vi "DAQ.Calibrate.vi"(8 "error in (no error)":errorcluster, 11 "Lockin.DAQ in":refnum<class "Instrument.DAQ.lvclass">) -> (0 "error out":errorcluster, 3 "Lockin.DAQ out":refnum<class "Instrument.DAQ.lvclass">)   [LabVIEW 2019, in "Instrument.Lockin.lvlib" / "Instrument.DAQ.lvclass"]
uses:
  Instrument.DAQ.lvclass
  DAQmx/typedefs/DAQmx.Commands--enum.ctl
  Instrument.DAQ.lvclass/Instrument.DAQ.ctl
  DAQmx/DAQmx.lvclass
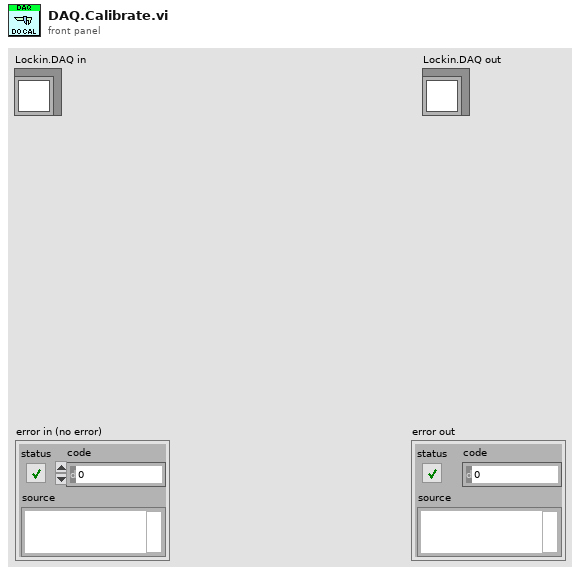
[diagram p1: front panel]
types:
  T1 = typedef "DAQmx.lvclass/DAQmx.Commands--enum.ctl" = enum16{"idle", "start", "stop", "calibrate", "auto", "exit"}
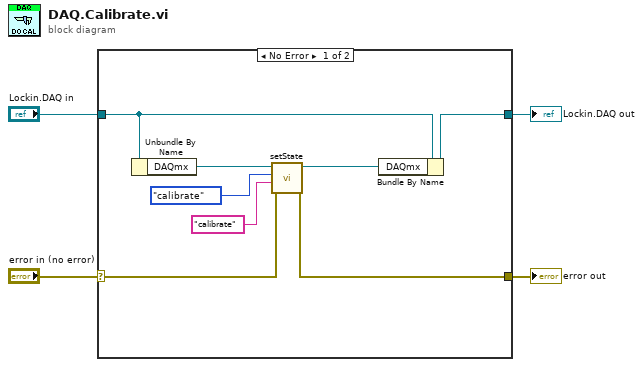
[diagram p0: block diagram]
diagram:
  n1 = case shown="No Error" "error in (no error)" {
    selector: "error in (no error)" -> [w7 w14]
    tunnel: [w11 w13] -> w4
    tunnel: [w6 w14] -> w3
    tunnel: "Lockin.DAQ in" -> [w12 w13]
    frame No Error {
      n2 = Unbundle By Name(w12) -> ("DAQmx"=w9:refnum<class "DAQmx.lvclass">)
      n3 = call "setState.vi"("error in (no error)"=w7, "Argument"="calibrate", "Command"=DAQmx.Commands--enum."calibrate" ("State"), "DAQmx in"=w9) -> ("error out"=w6:errorcluster, "DAQmx out"=w8:refnum<class "DAQmx.lvclass">)  [unwired: 6 in]
      n4 = Bundle By Name(cluster=w12, "DAQmx"=w8) -> (w11:refnum<class "Instrument.DAQ.lvclass">)
    }
    frame Error {
    }
  }
  "error out" <- w3
  "Lockin.DAQ out" <- w4
